vi "Generate Return Param Info.vi"(11 "QObject Writer in":refnum<class "QObject Writer.lvclass">) -> (2 "Param Info":T1={"Parameter Name"="", "Num Dimensions"=1, "Parameter Type"=enum."Numeric", "Numeric Type"=enum."I32", "Param Passing"=enum."By Value", "Array Passing"=enum."Array Data Pointer", "String Passing"=enum."C String Pointer", "Adapt Format"=enum."By Value", "ActiveX Types"=enum."ActiveX Variant Pointer", "Const (unused)"=FALSE, "Minimum Size"=""}, 3 "QObject Writer out":refnum<class "QObject Writer.lvclass">)   [LabVIEW 2013, in "QObject Writer.lvclass"]
uses:
  QObject Writer.lvclass
  Data Structures/DLL Parameter Info.ctl
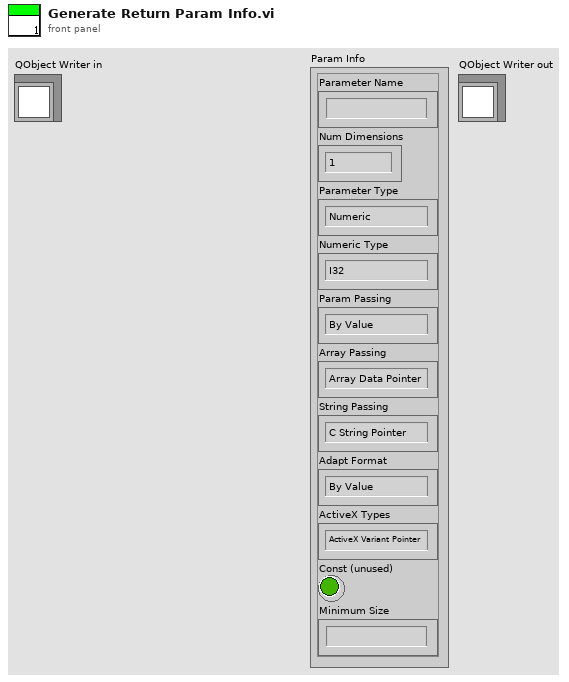
[diagram p1: front panel]
types:
  T1 = typedef "DLL Parameter Info.ctl" = cluster{"Parameter Name":string, "Num Dimensions":i32, "Parameter Type":enum16{"Numeric", "Array", "String", "Waveform", "Digital Waveform", "Digital Table", "ActiveX", "Any", "Instance Data Pointer", "Void"}, "Numeric Type":enum16{"I8", "I16", "I32", "I64", "U8", "U16", "U32", "U64", "SGL", "DBL", "PTR INT", "PTR UINT"}, "Param Passing":enum16{"By Value", "Pointer To Value"}, "Array Passing":enum16{"Array Data Pointer", "Array Handle", "Array Handle Pointer"}, "String Passing":enum16{"C String Pointer", "Pascal String Pointer", "String Handle", "String Handle Pointer"}, "Adapt Format":enum16{"By Value", "Pointer To Value"}, "ActiveX Types":enum16{"ActiveX Variant Pointer", "IDispatch* Pointer", "IUnknown* Pointer"}, "Const (unused)":bool, "Minimum Size":string}
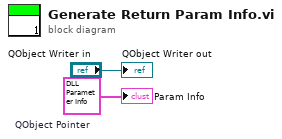
[diagram p0: block diagram]
diagram:
  w2 = T1 {"Parameter Name"="retVal", "Num Dimensions"=1, "Parameter Type"=enum."Numeric", "Numeric Type"=enum."U32", "Param Passing"=enum."Pointer To Value", "Array Passing"=enum."Array Data Pointer", "String Passing"=enum."C String Pointer", "Adapt Format"=enum."By Value", "ActiveX Types"=enum."ActiveX Variant Pointer", "Const (unused)"=FALSE, "Minimum Size"=""}  # QObject Pointer
  "QObject Writer out" <- "QObject Writer in"
  "Param Info" <- w2
